vi "PIDcontroDCmotorUsingMyRio.vi"() -> ()   [LabVIEW 2017]
uses:
  <vilib>/myRIO/Common/Instrument Driver Framework/myRIO v1.0/Encoder/typedefs/Encoder Count Direction Enum.ctl
  <vilib>/myRIO/Instrument Drivers/Onboard IO/Encoder/vis/Read.vi
  <vilib>/myRIO/Instrument Drivers/Onboard IO/PWM/vis/Set Duty Cycle and Frequency.vi
  <vilib>/myRIO/Instrument Drivers/Onboard IO/DIO/vis/Write.vi
  <vilib>/myRIO/Common/Instrument Driver Framework/myRIO v1.0/UART/vis/myRIO v1.0 Close UART.vi
  <vilib>/myRIO/Instrument Drivers/Onboard IO/Encoder/vis/Smart Open.vi
  <vilib>/Utility/error.llb/Error Cluster From Error Code.vi
  <vilib>/myRIO/Common/Instrument Driver Framework/myRIO v1.0/Encoder/vis/myRIO v1.0 Read Encoder.vi
  <vilib>/addons/control/pid/pid.llb/PID (DBL).vi
  <vilib>/myRIO/Instrument Drivers/Onboard IO/PWM/vis/Smart Open.vi
  <vilib>/myRIO/Common/Instrument Driver Framework/myRIO v1.0/PWM/vis/myRIO v1.0 Write PWM.vi
  <vilib>/myRIO/Instrument Drivers/Onboard IO/DIO/vis/Smart Open.vi
  <vilib>/myRIO/Common/Instrument Driver Framework/myRIO v1.0/DIO/vis/myRIO v1.0 Write DIO.vi
  <vilib>/myRIO/Common/Instrument Driver Framework/Utilities/vis/FPGA Ref Manager.vi
  <vilib>/myRIO/Common/Instrument Driver Framework/myRIO v1.0/myRIO v1.0 Reset FPGA.vi
  <vilib>/myRIO/Common/Instrument Driver Framework/myRIO v1.0/IRQ/vis/myRIO v1.0 IRQ Info FGV.vi
  <vilib>/myRIO/Common/Instrument Driver Framework/myRIO v1.0/IRQ/vis/myRIO v1.0 Timer IRQ Info FGV.vi
  <vilib>/myRIO/Common/Instrument Driver Framework/myRIO v1.0/IRQ/vis/myRIO v1.0 ISR Agent.vi
  <vilib>/myRIO/Instrument Drivers/Utilities/Utilities.lvlib
  <vilib>/addons/control/pid/NI_PID_pid.lvlib
panel:
  in  "PID gains":T1={"proportional gain (Kc)"=1.0, "integral time (Ti, min)"=0.01, "derivative time (Td, min)"=0.0} {"derivative time (Td, min)" format="%.3f"; "integral time (Ti, min)" format="%.3f"; "proportional gain (Kc)" format="%.3f"}
  out "Motor Speed":dbl(knob) caption="Gauge" scale=0.0..150.0
  out "Motor Response-SetSpeed vs. AcualSpeed":cluster{"Speed SetPoint":dbl, dbl}(graph)
  out "RPS":dbl
  out "RPM":dbl
  out "PPS":dbl
  out "Direction":bool
  in  "Enable":bool
  in  "Speed SetPoint":dbl(slide) scale=0.0..106.0
  in  "PWM freq [Hz]":dbl(slide)=100.0 scale=40.0..40000.0
  in  "Reset Counter":bool
  out "Counter Direction":T2
  out "Counter Value":i32
  in  "[ESC]":bool
  # "H-Bridge & Geared Motor demo Real Time control and Tuning using MyRio-1900"
  # "By Abdalrahman M. Amer \nabdalrahman.m5959@Gmail.com"
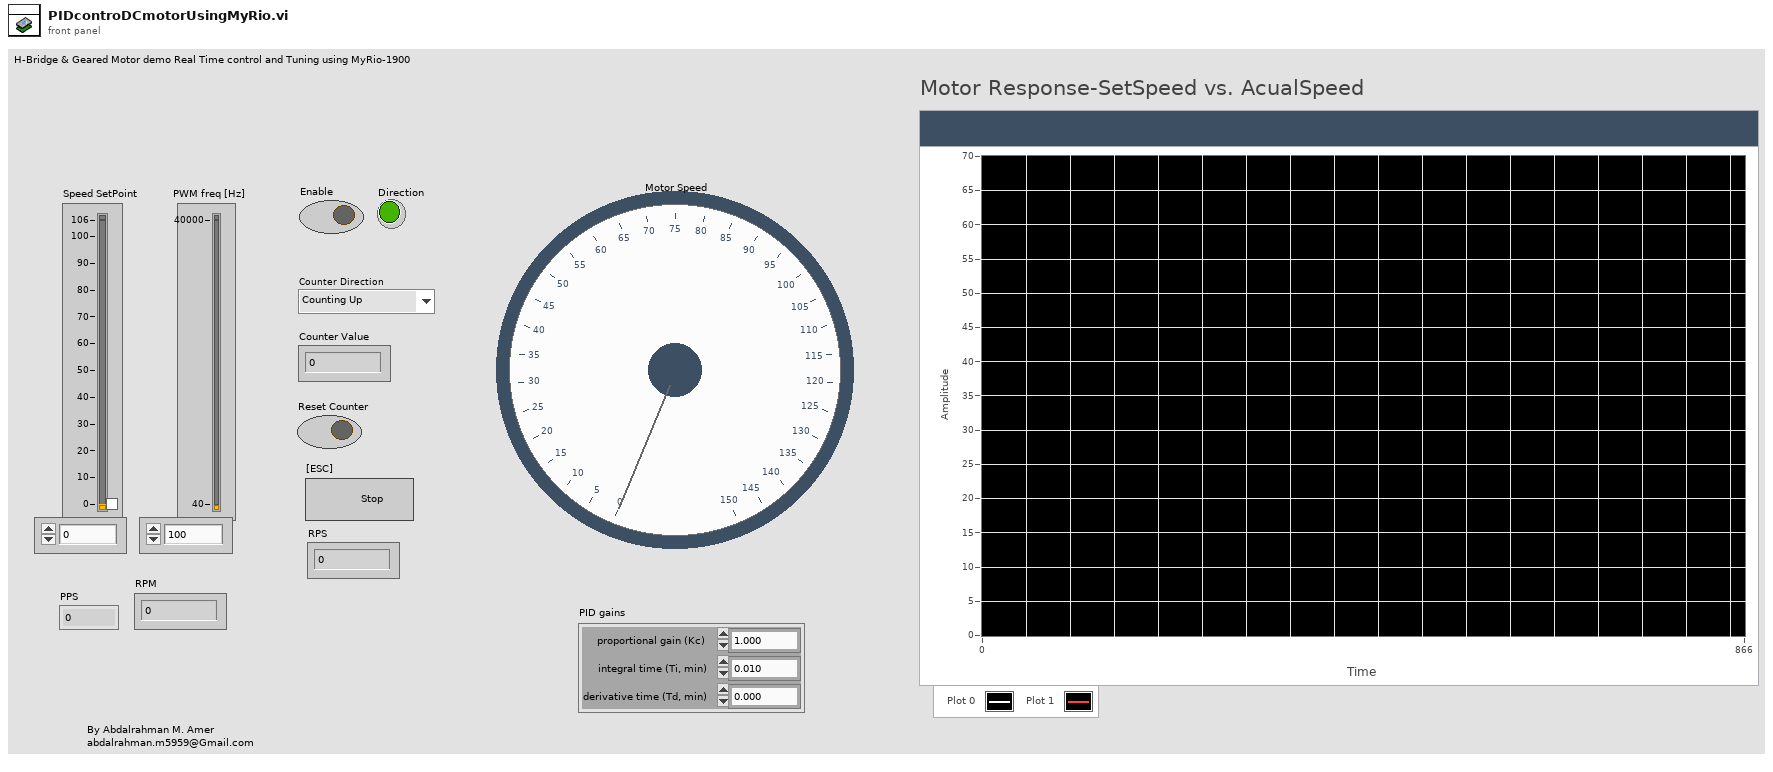
[diagram p1: front panel]
types:
  T1 = cluster{"proportional gain (Kc)":dbl, "integral time (Ti, min)":dbl, "derivative time (Td, min)":dbl}
  T2 = typedef "Encoder Count Direction Enum.ctl" = enum16{"Counting Up", "Counting Down"}
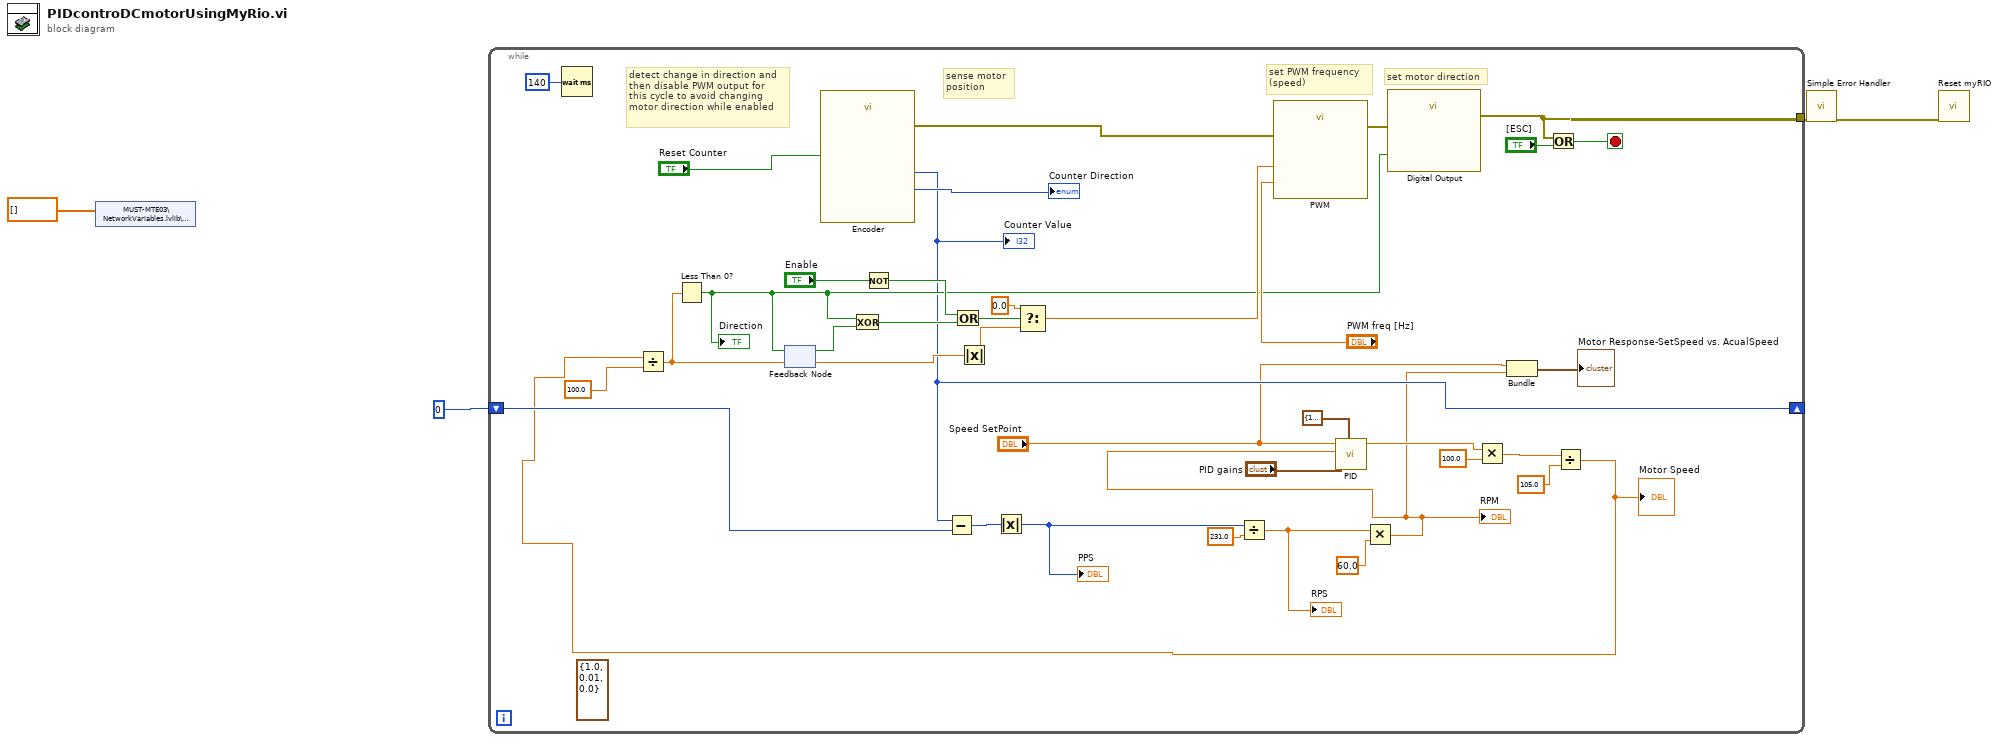
[diagram p0: block diagram]
diagram:
  n1 = shared-variable "MUST-MTE03\\NetworkVariables.lvlib\\RobotPath"(dbl[] [] ("RobotPath")) -> ()  [unwired: 1 in, 1 out]
  n2 = while {
    tunnel: [w33] -> w2
    shift-right: [w16] -> _
    shift-left: 0 ("Counter Value") -> [w17]
    stop <- w41 stop-if-true
    (unwired) T1 {"proportional gain (Kc)"=1.0, "integral time (Ti, min)"=0.01, "derivative time (Td, min)"=0.0} ("PID gains")
    # "sense motor \nposition"
    # "detect change in direction and\nthen disable PWM output for\nthis cycle to avoid changing\nmotor direction while enabled"
    # "set PWM frequency\n(speed)"
    # "set motor direction"
    n3 = Wait (ms)(milliseconds to wait=u32 140) -> ()  [unwired: 1 out]
    n4 = feedback #1() -> (w35:bool)  [unwired: 1 in]
    n5 = call "Encoder"("Reset Counter"="Reset Counter") -> ("Counter Value"=w16:i32, "Counter Direction"=→"Counter Direction":T2, "error out"=w37:errorcluster)  [unwired: 23 in, 1 out]
    "Counter Value" <- w16
    n6 = Not(x="Enable") -> (.not. x?=w29:bool)
    n7 = Subtract(x=w16, y=w17) -> (x-y=w15:i32)
    n8 = Absolute Value(x=w15) -> (abs(x)=w21:i32)
    "PPS" <- w21
    n9 = Divide(x=w21, y=231.0) -> (x/y=w18:dbl)
    "RPS" <- w18
    n10 = Multiply(x=w18, y=60.0) -> (x*y=w9:dbl)
    "RPM" <- w9
    n11 = call-poly <vilib>:"PID.vi"("output range"=cluster{"output high":dbl, "output low":dbl} {"output high"=106.0, "output low"=0.0}, "PID gains"="PID gains", "process variable"=w9, "setpoint"="Speed SetPoint") -> ("output"=w13:dbl)  [unwired: 6 in, 1 out]
    n12 = Multiply(x=w13, y=100.0) -> (x*y=w14:dbl)
    n13 = Bundle("Speed SetPoint"="Speed SetPoint", w9) -> (→"Motor Response-SetSpeed vs. AcualSpeed":cluster{"Speed SetPoint":dbl, dbl})  [unwired: 1 in]
    n14 = Divide(x=w14, y=105.0) -> (x/y=w6:dbl)
    "Motor Speed" <- w6
    n15 = Divide(x=w6, y=100.0) -> (x/y=w26:dbl)
    n16 = Less Than 0?(x=w26) -> (x < 0?=w23:bool)
    "Direction" <- w23
    n17 = feedback-in #1(w23) -> ()
    n18 = Exclusive Or(1:w35, 2:w23) -> (0:w32:bool)
    n19 = Or(x=w29, y=w32) -> (x .or. y?=w31:bool)
    n20 = Absolute Value(x=w26) -> (abs(x)=w24:dbl)
    n21 = Select(t=0.0 ("f"), s=w31, f=w24) -> (s? t:f=w25:dbl)
    n22 = call "PWM"("Duty Cycle"=w25, "Frequency [Hz]"="PWM freq [Hz]", "error in (no error)"=w37) -> ("error out"=w36:errorcluster)  [unwired: 24 in]
    n23 = call "Digital Output"("A/DIO0 (Pin 11)"=w23, "error in (no error)"=w36) -> ("error out"=w33:errorcluster)  [unwired: 25 in]
    n24 = Or(x=w33, y="[ESC]") -> (x .or. y?=w41:bool)
  }
  n25 = call <vilib>:"Simple Error Handler.vi"("error in (no error)"=w2) -> ("error out"=w3:errorcluster)  [unwired: 4 in, 4 out]
  n26 = call <vilib>:"Reset myRIO.vi"("error in (no error)"=w3) -> ()  [unwired: 10 in, 1 out]
